vi "LVFunction_Imop_HAS file_GetAcquisitionInformation.vi"(0 "HAS file path":path, 11 "error in (no error)":errorcluster) -> (6 "HAS file information":T1, 15 "error out":errorcluster)   [LabVIEW 2020]
doc: "Get informations from .has file.\n\n--------------------------------------------------------------------------------\n\n<B>has_file_pathIn</B> : Absolute path to the .has file.\n\n<B>has_file_pathOut</B> : Absolute path to the .has file.\n\n<B>haso_model</B> : Haso Sensor model.\n\n<B>haso_serial_number</B> : Haso Serial number.\n\n<B>revision</B> : Revision number.\n\n<B>size</B> : HasoData dimension (subpupil number)\n\n<B>step</B> : HasoData sampling step (um).\n\n<B>time_stamp</B> : Timestamp.\n\n<B>comments</B> : Comments\n\n<B>session_name</B> : Session name.\n\n<B>wavelength_nm</B> : Source wavelength (nm).\n\n<B>lower_calibration_wl</B> : Lower calibration wavelength (nm).\n\n<B>upper_calibration_wl</B> : Upper calibration wavelength (nm).\n\n<B>ErrorIn</B> : Error\n\n<B>ErrorOut</B> : Error"
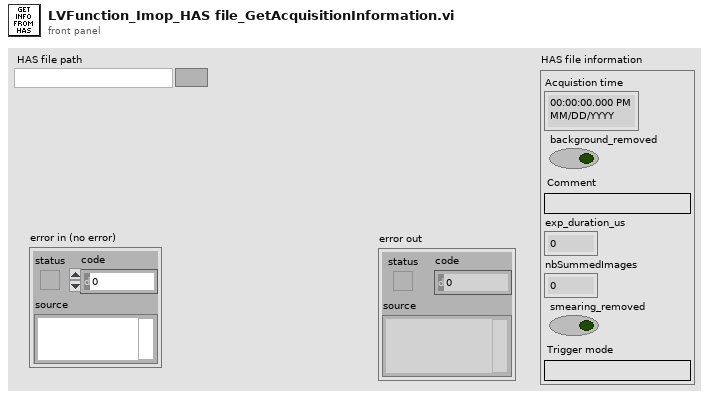
[diagram p1: front panel]
types:
  T1 = cluster{"Acquistion time":timestamp, "background_removed":bool, "Comment":string, "exp_duration_us":u32, "nbSummedImages":u32, "smearing_removed":bool, "Trigger mode":string}
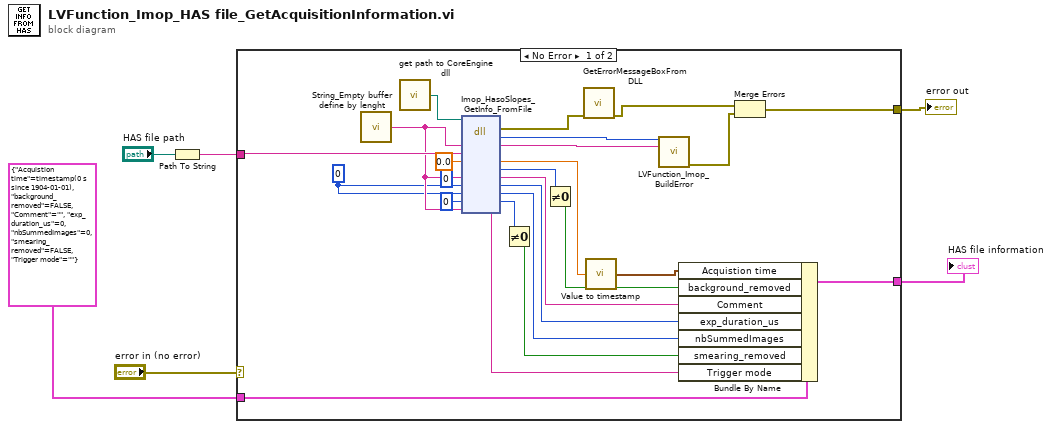
[diagram p0: block diagram]
diagram:
  n1 = Path To String(path="HAS file path") -> (string=w3:string)
  n2 = case shown="No Error" "error in (no error)" {
    selector: "error in (no error)" -> [_ w32]
    tunnel: [w20 w32] -> w5
    tunnel: w3 -> [w27 _]
    tunnel: T1 {"Acquistion time"=timestamp(0 s since 1904-01-01), "background_removed"=FALSE, "Comment"="", "exp_duration_us"=0, "nbSummedImages"=0, "smearing_removed"=FALSE, "Trigger mode"=""} ("HAS file information") -> [w26 _]
    tunnel: [w25 _] -> w2
    frame No Error {
      w9 = u32 0 ("Revision")
      n3 = call "String_Empty buffer define by lenght.vi"() -> ("Empty buffer"=w13:string)  [unwired: 1 in]
      n4 = call "get path to CoreEngine dll.vi"() -> ("path to wavekit library"=w29:path)  [unwired: 14 in, 1 out]
      n5 = dll-call lib="D:/2_trunk/Soft_haso/ImOpCoreEngine4_LV2011/DLLs/ImopEngine4_vc100.dll" fn="Imop_HasoSlopes_GetInfo_FromFile"(path in=w29, "message"=w13, "HasFilePath"=w27, "TimeStamp"=0.0, "background_removed"=u8 0, "comment"=w13, "exp_duration_us"=w9, "nbSummedImages"=w9, "smearing_removed"=u8 0, "trigger_mode"=w13) -> (error out=w28:errorcluster, "return type"=w31:i32, "message"=w30:string, "TimeStamp"=w19:dbl, "background_removed"=w18:u8, "comment"=w23:string, "exp_duration_us"=w15:u32, "nbSummedImages"=w14:u32, "smearing_removed"=w17:u8, "trigger_mode"=w12:string)  [unwired: 3 in, 1 out]
      n6 = Not Equal To 0?(x=w17) -> (x != 0?=w11:bool)
      n7 = Not Equal To 0?(x=w18) -> (x != 0?=w16:bool)
      n8 = call "GetErrorMessageBoxFromDLL.vi"("error IN"=w28) -> ("error OUT"=w22:errorcluster)  [unwired: 10 in]
      n9 = call "Value to timestamp.vi"("TimeStamp"=w19) -> ("Time Stamp"=w24:timestamp)
      n10 = call "LVFunction_Imop_BuildError.vi"("code"=w31, "String to Prepend to source (\"\")"=w30) -> ("error out"=w21:errorcluster)  [unwired: 13 in]
      n11 = Bundle By Name(cluster=w26, "Acquistion time"=w24, "background_removed"=w16, "Comment"=w23, "exp_duration_us"=w15, "nbSummedImages"=w14, "smearing_removed"=w11, "Trigger mode"=w12) -> (w25:T1)
      n12 = Merge Errors(w22, w21) -> (w20:errorcluster)
    }
    frame Error {
    }
  }
  "error out" <- w5
  "HAS file information" <- w2
